vi "Globales.vi"() -> ()   [LabVIEW 2017]
panel:
  in  "Avance_Calibrar":dbl
  in  "RangoY":dbl
  out "PosY":dbl
  out "RelY":dbl
  out "MoveY":bool
  in  "RangoX":dbl
  out "PosX":dbl
  out "RelX":dbl
  out "MoveX":bool
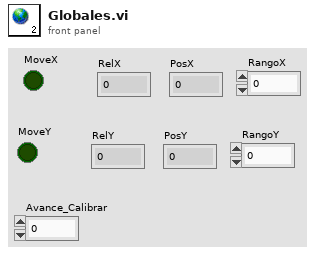
[diagram p1: front panel]
diagram:
